vi "Periodic Tasks.vi"(8 "error in":errorcluster) -> ()   [LabVIEW 2014]
doc: "This VI runs in parallel to other tasks. It can contain as many user-defined periodic loops as you need. These can carry out PID or other sorts of timed response."
uses:
  <vilib>/Rock Robotics/SystemInterfaces/Utilities/FPGA_UtilitiesLED Source.ctl
  <vilib>/Rock Robotics/SystemInterfaces/Utilities/FPGA_UtilitiesLED State.ctl
  Robot Global Data.vi
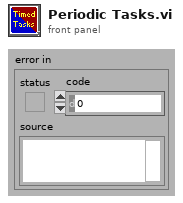
[diagram p1: front panel]
types:
  T1 = typedef "FPGA_UtilitiesLED State.ctl" = enum16{"Off", "On", "Toggle"}
  T2 = typedef "FPGA_UtilitiesLED Source.ctl" = enum16{"User LED", "FPGA LED"}
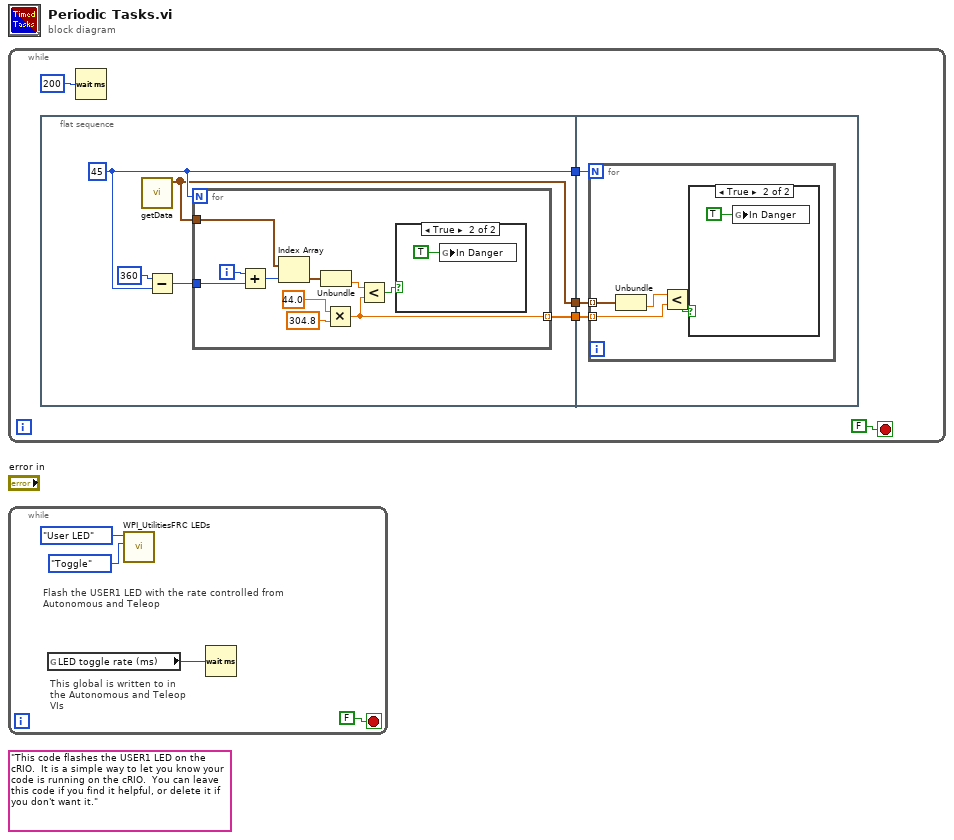
[diagram p0: block diagram]
diagram:
  (unwired) "This code flashes the USER1 LED on the cRIO.  It is a simple way to let you know your code is running on the cRIO.  You can leave this code if you find it helpful, or delete it if you don't want it."
  n1 = while {
    stop <- FALSE stop-if-true
    n2 = flat-sequence {
      tunnel: [w8] -> w3
      tunnel: [w7] -> w2
      tunnel: [w6] -> w1
      tunnel: w3 -> [w24]
      tunnel: w2 -> [w23]
      tunnel: w1 -> [w22]
      frame #0 {
        w8 = 45
        n3 = call "getData.vi"() -> ("output array"=w6:cluster{"Degree":dbl, "Magnitude":dbl}[])  [unwired: 11 in]
        n4 = Subtract(x=360, y=w8) -> (x-y=w9:i32)
        n5 = for {
          N: w8 -> [_]
          tunnel: w6 -> [w19]
          tunnel: w9 -> [w16]
          tunnel: [w12] -> w7 mode=indexing
          i -> [w18]
          n6 = Add(x=w18, y=w16) -> (x+y=w17:i32)
          n7 = Index Array(array=w19, index=w17) -> (element=w20:cluster{"Degree":dbl, "Magnitude":dbl})
          n8 = Unbundle(w20) -> ("Magnitude"=w13:dbl)  [unwired: 1 out]
          n9 = Multiply(x=44.0, y=304.8) -> (x*y=w12:dbl)
          n10 = Less?(x=w13, y=w12) -> (x < y?=w11:bool)
          n11 = case shown="True" w11 {
            frame False {
            }
            frame True {
              n12 = global write "Robot Global Data.vi" "In Danger"(TRUE) -> ()
            }
          }
        }
      }
      frame #1 {
        n13 = for {
          N: w24 -> [_]
          tunnel: w22 -> [w28] mode=indexing
          tunnel: w23 -> [w27] mode=indexing
          n14 = Unbundle(w28) -> ("Magnitude"=w25:dbl)  [unwired: 1 out]
          n15 = Less?(x=w25, y=w27) -> (x < y?=w26:bool)
          n16 = case shown="True" w26 {
            frame False {
            }
            frame True {
              n17 = global write "Robot Global Data.vi" "In Danger"(TRUE) -> ()
            }
          }
        }
      }
    }
    n18 = Wait (ms)(milliseconds to wait=u32 200) -> ()  [unwired: 1 out]
  }
  n19 = while {
    stop <- FALSE stop-if-true
    # "This global is written to in the Autonomous and Teleop VIs"
    # "Flash the USER1 LED with the rate controlled from Autonomous and Teleop"
    n20 = global read "Robot Global Data.vi" "LED toggle rate (ms)"() -> (w30:u32)
    n21 = call <vilib>:"WPI_UtilitiesFRC LEDs.vi"("State"=FPGA_UtilitiesLED_State."Toggle", "LED Type"=FPGA_UtilitiesLED_Source."User LED") -> ()  [unwired: 1 in, 9 out]
    n22 = Wait (ms)(milliseconds to wait=w30) -> ()  [unwired: 1 out]
  }
